vi "Determine FAxial FLateral Force.vi"(8 "error in (no error)":errorcluster, 9 "FC2":dbl[unit], 10 "FC1":dbl[unit], 11 "Model in":refnum<class "Model.lvclass">) -> (0 "error out":errorcluster, 1 "Lateral Force":dbl[unit], 2 "Axial Force":dbl[unit], 3 "Model out":refnum<class "Model.lvclass">)   [LabVIEW 2015, in "Model.lvclass"]
uses:
  Model.lvclass
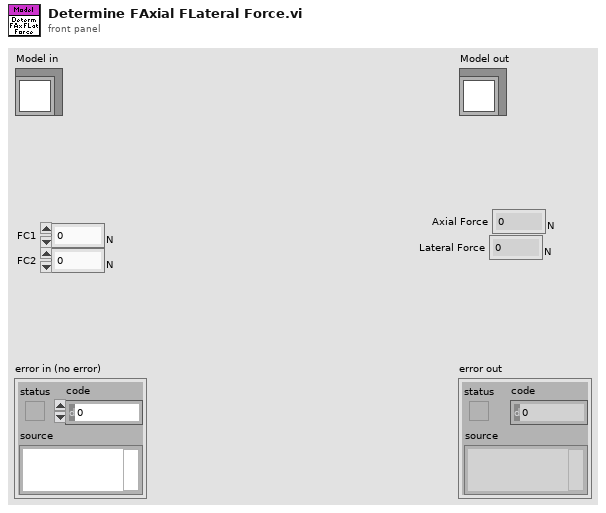
[diagram p1: front panel]
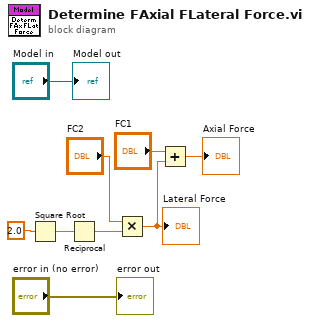
[diagram p0: block diagram]
diagram:
  n1 = Square Root(x=2.0) -> (sqrt(x)=w3:dbl)
  n2 = Reciprocal(x=w3) -> (1/x=w2:dbl)
  n3 = Multiply(x="FC2", y=w2) -> (x*y=w6:dbl[unit])
  "Lateral Force" <- w6
  n4 = Add(x="FC1", y=w6) -> (x+y=→"Axial Force":dbl[unit])
  "error out" <- "error in (no error)"
  "Model out" <- "Model in"
